vi "DAQ-WriteValue.vi"(6 "Input":dbl format="%0.2f", 8 "DAQ?":bool, 9 "DAQ Device IN":T1={"DAQ Fs (S/s)"=10000.0, "task"="", "error"={"status"=FALSE, "code"=0, "source"=""}, "Min Value"=-10.0, "Max Value"=10.0}) -> (2 "In Range?":bool, 3 "DAQ Device OUT":T1={"DAQ Fs (S/s)"=0.0, "task"="", "error"={"status"=FALSE, "code"=0, "source"=""}, "Min Value"=-10.0, "Max Value"=10.0})   [LabVIEW 2010]
uses:
  <vilib>/DAQmx/write.llb/DAQmx Write (Analog DBL 1Chan 1Samp).vi
  <vilib>/daqmx/miscellaneous.llb/DAQmx Fill In Error Info.vi
panel:
  out "#samples out":u32
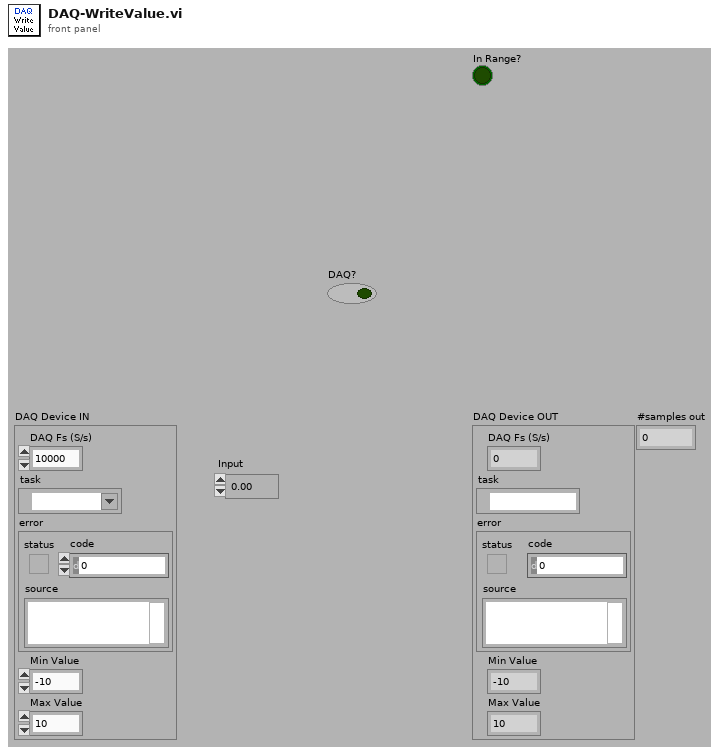
[diagram p1: front panel]
types:
  T1 = cluster{"DAQ Fs (S/s)":dbl, "task":refnum<k21>, "error":errorcluster, "Min Value":dbl, "Max Value":dbl}
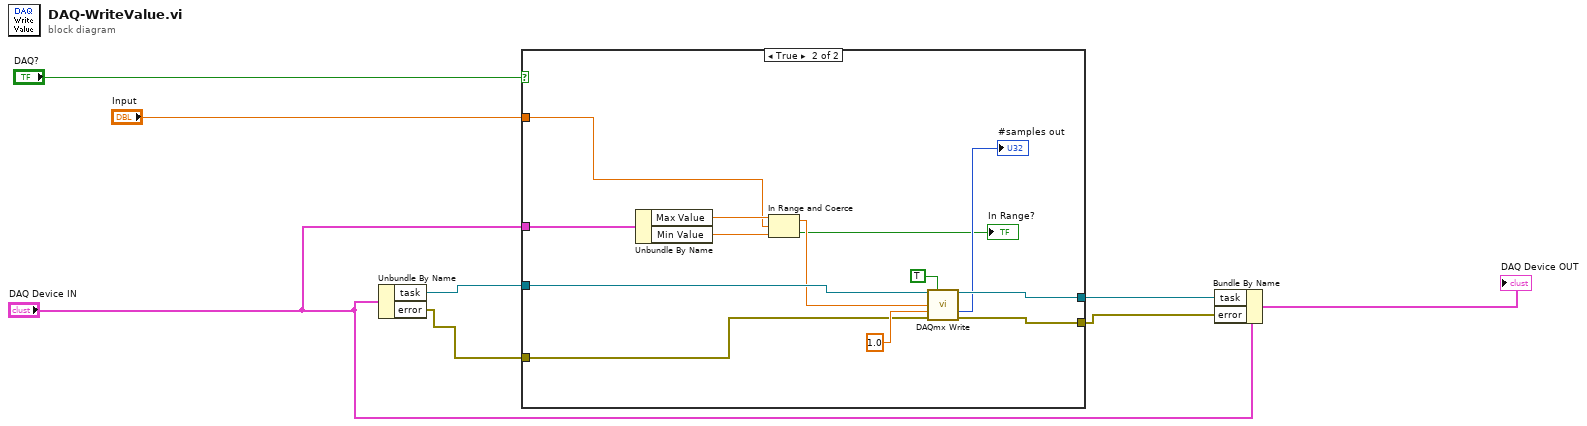
[diagram p0: block diagram]
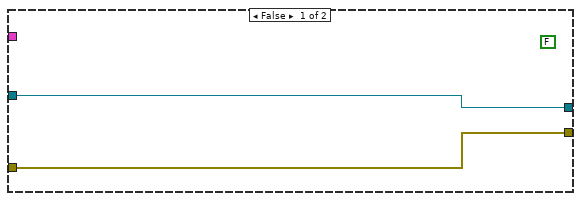
[diagram p2: hidden frame]
diagram:
  n1 = Unbundle By Name("DAQ Device IN") -> ("task"=w6:refnum<k21>, "error"=w2:errorcluster)
  n2 = case shown="True" "DAQ?" {
    tunnel: w6 -> [w9 w18]
    tunnel: [w9 w23] -> w4
    tunnel: w2 -> [w10 w17]
    tunnel: [w10 w22] -> w5
    tunnel: "Input" -> [_ w13]
    tunnel: "DAQ Device IN" -> [_ w14]
    frame False {
      (unwired) FALSE
    }
    frame True {
      n3 = Unbundle By Name(w14) -> ("Max Value"=w15:dbl, "Min Value"=w16:dbl)
      n4 = In Range and Coerce(upper limit=w15, x=w13, lower limit=w16) -> (coerced(x)=w12:dbl, In Range?=→"In Range?":bool)
      n5 = call-poly <vilib>:"DAQmx Write.vi"("task/channels in"=w18, "auto start"=TRUE, "data"=w12, "timeout"=1.0, "error in"=w17) -> ("task out"=w23:refnum<k21>, "number of samples written per channel"=→"#samples out":u32, "error out"=w22:errorcluster)  [unwired: 8 in]
    }
  }
  n6 = Bundle By Name(cluster="DAQ Device IN", "task"=w4, "error"=w5) -> (→"DAQ Device OUT":T1)
